vi "relative access path.vi"(11 "Oauth2.GitLab":refnum<class "Oauth2.GitLab.lvclass">) -> (1 "Token Access Path":string, 2 "Authorization Path":string)   [LabVIEW 2013, in "Oauth2.GitLab.lvclass"]
uses:
  Oauth2.GitLab.lvclass
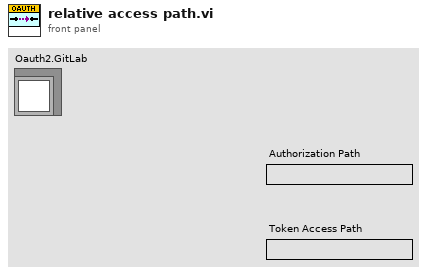
[diagram p1: front panel]
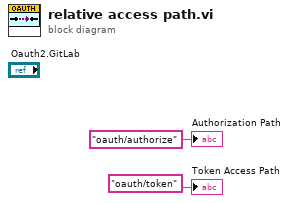
[diagram p0: block diagram]
diagram:
  "Authorization Path" <- "oauth/authorize" ("Authorization Path")
  "Token Access Path" <- "oauth/token" ("Authorization Path")
